vi "Build DashBoard Data.vi"() -> ()   [LabVIEW 2011]
doc: "This VI builds data and sends it back to the dashboard PC program. By default it sends back the raw values for the first analog, digital, and solenoid module. Modify it to send back the data you want to view. Consider adding higher level data to the Dashboard Datatype.ctl and to this VI. Then update the Dashboard to display the data however you like.\n\nThis software is licensed. Open the labview\\readme\\WPI Robotics Library Open Source License.txt file for more information."
uses:
  Shared/Dashboard Datatype.ctl
  Shared/Drive Base Dashboard Package.ctl
  Shared/Shifter State.ctl
  Shared/Shooter Dashboard Package.ctl
  Shared/Shooter Control Mode.ctl
  Shared/cRIO Performance Details.ctl
  Robot Global Data.vi
  Shooter Global.vi
panel:
  out "Dashboard Data":T1={"Drive Base"={"Left"=0.0, "Right"=0.0, "Shifter"=enum."Unknown"}, "Shooter"={"Set RPM"=0.0, "Current RPM"=0.0, "Motor Speed"=0.0, "Shooter Mode"=enum."Off", "Shooter Speed Enumerated Type"=enum."Off"}, "Performance Details"={"CPU Utilization"=0.0, "RAM total (bytes)"=0, "RAM available (bytes)"=0, "Flash size (bytes)"=0, "Flash free (bytes)"=0}} {"Performance Details"."CPU Utilization" format="%#.2f"}
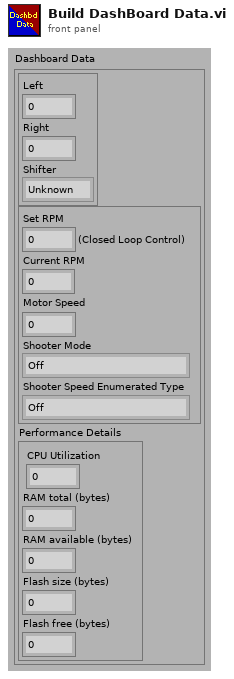
[diagram p1: front panel]
types:
  T1 = typedef "Dashboard Datatype.ctl" = cluster{"Drive Base":T2, "Shooter":T4, "Performance Details":T6}
  T2 = typedef "Drive Base Dashboard Package.ctl" = cluster{"Left":dbl, "Right":dbl, "Shifter":T3}
  T3 = typedef "Shifter State.ctl" = enum16{"Unknown", "Low", "High"}
  T4 = typedef "Shooter Dashboard Package.ctl" = cluster{"Set RPM":dbl, "Current RPM":dbl, "Motor Speed":dbl, "Shooter Mode":enum16{"Off", "Open Loop Control", "Closed Loop Control", "Top Spin"}, "Shooter Speed Enumerated Type":T5}
  T5 = typedef "Shooter Control Mode.ctl" = enum16{"Key", "Mid Field", "Backfield", "Topspin", "Open Loop Control", "Off"}
  T6 = typedef "cRIO Performance Details.ctl" = cluster{"CPU Utilization":dbl, "RAM total (bytes)":u32, "RAM available (bytes)":u32, "Flash size (bytes)":i64, "Flash free (bytes)":i64}
  T7 = enum16{"Off", "Open Loop Control", "Closed Loop Control", "Top Spin"}
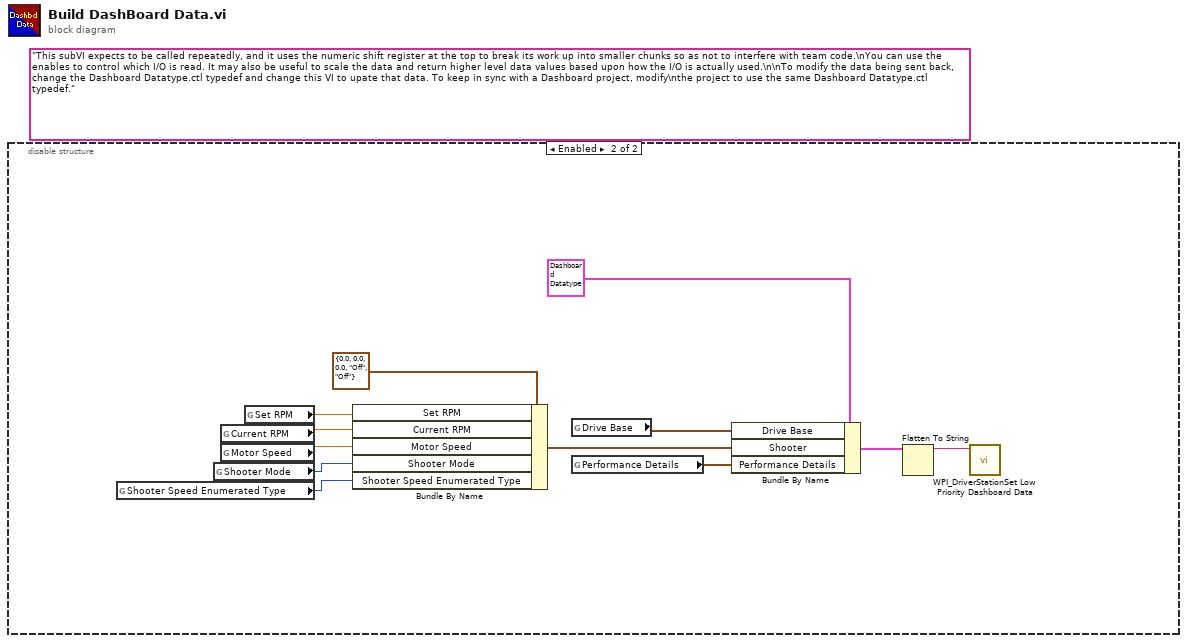
[diagram p0: block diagram]
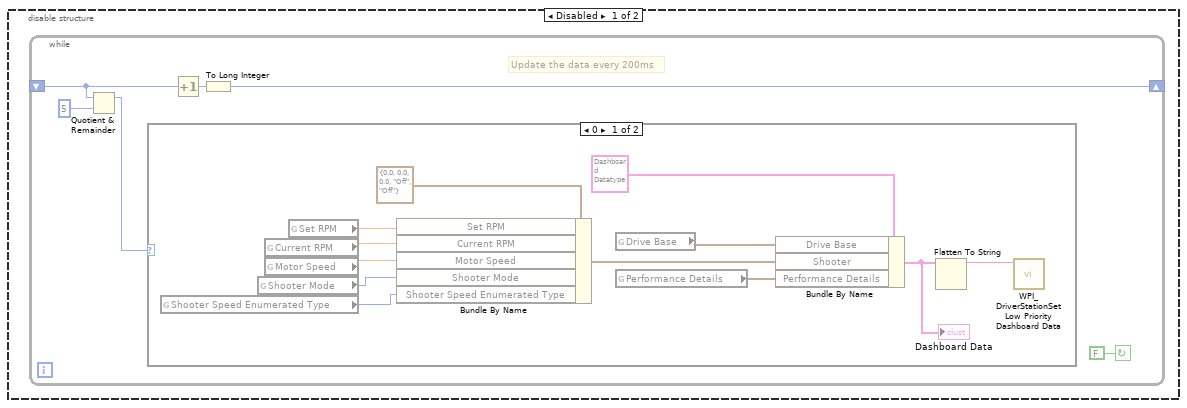
[diagram p2: hidden frame]
diagram:
  (unwired) "This subVI expects to be called repeatedly, and it uses the numeric shift register at the top to break its work up into smaller chunks so as not to interfere with team code.\nYou can use the enables to control which I/O is read. It may also be useful to scale the data and return higher level data values based upon how the I/O is actually used.\n\nTo modify the data being sent back, change the Dashboard Datatype.ctl typedef and change this VI to upate that data. To keep in sync with a Dashboard project, modify\nthe project to use the same Dashboard Datatype.ctl typedef."
  n1 = disable-structure shown="Enabled" {
    frame Disabled {
      n2 = while {
        shift-right: [w2] -> _
        shift-left: _ -> [w3]
        stop <- FALSE continue-if-true
        # "Update the data every 200ms"
        n3 = Quotient & Remainder(x=w3, y=5) -> (x-y*floor(x/y)=w1:i32)  [unwired: 1 out]
        n4 = case shown="0" w1 {
          frame 0 {
            n5 = global read "Shooter Global.vi" "Shooter Speed Enumerated Type"() -> (w9:T5)
            n6 = global read "Shooter Global.vi" "Shooter Mode"() -> (w10:T7)
            n7 = global read "Shooter Global.vi" "Current RPM"() -> (w12:dbl)
            n8 = global read "Shooter Global.vi" "Motor Speed"() -> (w11:dbl)
            n9 = global read "Shooter Global.vi" "Set RPM"() -> (w13:dbl)
            n10 = Bundle By Name(cluster=T4 {"Set RPM"=0.0, "Current RPM"=0.0, "Motor Speed"=0.0, "Shooter Mode"=enum."Off", "Shooter Speed Enumerated Type"=enum."Off"} ("Shooter"), "Set RPM"=w13, "Current RPM"=w12, "Motor Speed"=w11, "Shooter Mode"=w10, "Shooter Speed Enumerated Type"=w9) -> (w14:T4)
            n11 = global read "Robot Global Data.vi" "Drive Base"() -> (w16:T2)
            n12 = global read "Robot Global Data.vi" "Performance Details"() -> (w8:T6)
            n13 = Bundle By Name(cluster=T1 {"Drive Base"={"Left"=0.0, "Right"=0.0, "Shifter"=enum."Unknown"}, "Shooter"={"Set RPM"=0.0, "Current RPM"=0.0, "Motor Speed"=0.0, "Shooter Mode"=enum."Off", "Shooter Speed Enumerated Type"=enum."Off"}, "Performance Details"={"CPU Utilization"=0.0, "RAM total (bytes)"=0, "RAM available (bytes)"=0, "Flash size (bytes)"=0, "Flash free (bytes)"=0}} ("Dashboard Data"), "Drive Base"=w16, "Shooter"=w14, "Performance Details"=w8) -> (w7:T1)
            "Dashboard Data" <- w7
            n14 = Flatten To String(anything=w7) -> (data string=w18:string)  [unwired: 1 in, 4 out]
            n15 = call <vilib>:"WPI_DriverStationSet Low Priority Dashboard Data.vi"("User Data"=w18) -> ()  [unwired: 1 in, 10 out]
          }
          frame Default {
          }
        }
        n16 = Increment(x=w3) -> (x+1=w6:i32)
        n17 = To Long Integer(number=w6) -> (32bit integer=w2:i32)
      }
    }
    frame Enabled {
      n18 = global read "Shooter Global.vi" "Shooter Speed Enumerated Type"() -> (w19:T5)
      n19 = global read "Shooter Global.vi" "Shooter Mode"() -> (w22:T7)
      n20 = global read "Shooter Global.vi" "Current RPM"() -> (w24:dbl)
      n21 = global read "Shooter Global.vi" "Motor Speed"() -> (w23:dbl)
      n22 = global read "Shooter Global.vi" "Set RPM"() -> (w25:dbl)
      n23 = Bundle By Name(cluster=T4 {"Set RPM"=0.0, "Current RPM"=0.0, "Motor Speed"=0.0, "Shooter Mode"=enum."Off", "Shooter Speed Enumerated Type"=enum."Off"} ("Shooter"), "Set RPM"=w25, "Current RPM"=w24, "Motor Speed"=w23, "Shooter Mode"=w22, "Shooter Speed Enumerated Type"=w19) -> (w26:T4)
      n24 = global read "Robot Global Data.vi" "Drive Base"() -> (w28:T2)
      n25 = global read "Robot Global Data.vi" "Performance Details"() -> (w21:T6)
      n26 = Bundle By Name(cluster=T1 {"Drive Base"={"Left"=0.0, "Right"=0.0, "Shifter"=enum."Unknown"}, "Shooter"={"Set RPM"=0.0, "Current RPM"=0.0, "Motor Speed"=0.0, "Shooter Mode"=enum."Off", "Shooter Speed Enumerated Type"=enum."Off"}, "Performance Details"={"CPU Utilization"=0.0, "RAM total (bytes)"=0, "RAM available (bytes)"=0, "Flash size (bytes)"=0, "Flash free (bytes)"=0}} ("Dashboard Data"), "Drive Base"=w28, "Shooter"=w26, "Performance Details"=w21) -> (w20:T1)
      n27 = Flatten To String(anything=w20) -> (data string=w30:string)  [unwired: 1 in, 4 out]
      n28 = call <vilib>:"WPI_DriverStationSet Low Priority Dashboard Data.vi"("User Data"=w30) -> ()  [unwired: 1 in, 10 out]
    }
  }
